vi "Stop Core.vi"(10 "final error code":i32, 11 "Capillary Line in":refnum<class "Capillary Line.lvclass">) -> (3 "Capillary Line out":refnum<class "Capillary Line.lvclass">)   [LabVIEW 2015, in "cRIO-Carbondioxide.lvlib" / "CO2-Actor.lvlib" / "Capillary Line.lvclass"]
doc: "(<B>Filename</B>: Actor Framework.lvlib:Actor.lvclass:Stop Core.vi)\n\nDefines what the actor does before it stops. Use the <B>final error code</B> input to determine whether the actor shut down in response to an error.\n\nBy default, this method does nothing. A descendant class may override it to define behavior, such as shutting down any processes the actor initiated in its override of the Actor Core method."
uses:
  Capillary Line.lvclass
  Capillary Line.lvclass/Capillary Line.ctl
  CO2 Actor/CO2 Actor.lvclass
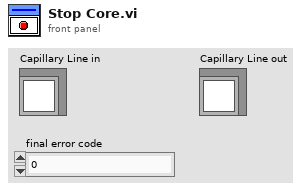
[diagram p1: front panel]
types:
  T1 = typedef "Sample Container.ctl" = cluster{"Sample In":refnum<k21>, "Sample Name":refnum<k21>, "Ti Cathode":refnum<k21>, "SampleQ":refnum<queue>}
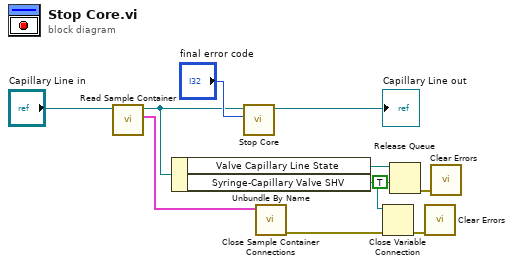
[diagram p0: block diagram]
diagram:
  n1 = call "Read Sample Container.vi"("Capillary Line in"="Capillary Line in") -> ("Container"=w8:T1, "Capillary Line out"=w7:refnum<class "Capillary Line.lvclass">)  [unwired: 7 in, 2 out]
  n2 = Unbundle By Name(w7) -> ("Valve Capillary Line State"=w3:refnum<queue>, "Syringe-Capillary Valve SHV"=w6:refnum<k21>)
  n3 = call-parent "Stop Core.vi"("final error code"="final error code", "CO2 Actor in"=w7) -> ("CO2 Actor out"=→"Capillary Line out":refnum<class "Capillary Line.lvclass">)  [unwired: 9 in]
  n4 = call "Close Sample Container Connections.vi"("Container in"=w8) -> ("error out"=w5:errorcluster)  [unwired: 9 in, 1 out]
  n5 = Close Variable Connection(8:w5, 11:w6) -> (0:w4:errorcluster)
  n6 = Release Queue(queue=w3, force destroy? (F)=TRUE) -> (error out=w2:errorcluster)  [unwired: 1 in, 2 out]
  n7 = call <vilib>:"Clear Errors.vi"("error in (no error)"=w4) -> ()  [unwired: 5 in, 2 out]
  n8 = call <vilib>:"Clear Errors.vi"("error in (no error)"=w2) -> ()  [unwired: 5 in, 2 out]
